vi "OEE_SCREEN_2_show_label_for_graphics.vi"(10 "Y_annotation_offset":dbl, 11 "values":cluster{dbl[], dbl[]}) -> (3 "annotations":T1(array[cluster]))   [LabVIEW 2020]
uses:
  <vilib>/Analysis/baseanly.llb/Mean (DBL).vi
  <vilib>/Analysis/NI_AALBase.lvlib
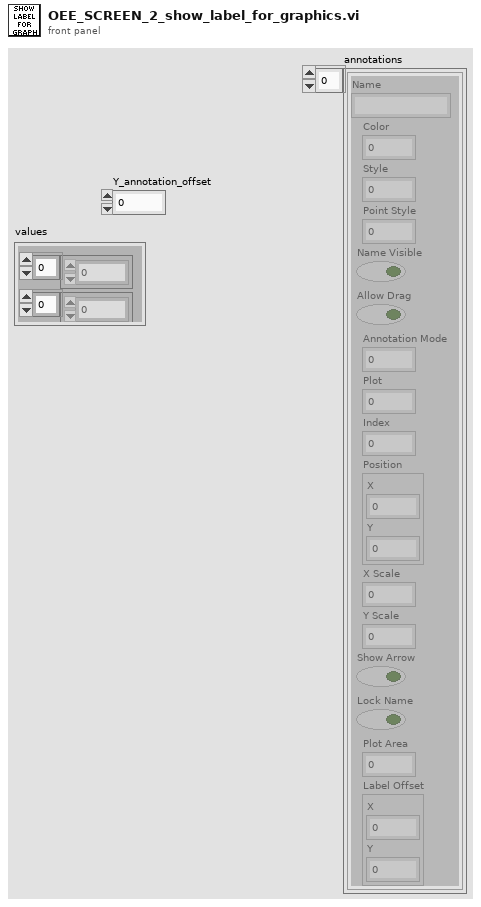
[diagram p1: front panel]
types:
  T1 = cluster{"Name":string, "Color":u32, "Style":u8, "Point Style":u8, "Name Visible":bool, "Allow Drag":bool, "Annotation Mode":u32, "Plot":i32, "Index":i32, "Position":cluster{"X":dbl, "Y":dbl}, "X Scale":u32, "Y Scale":u32, "Show Arrow":bool, "Lock Name":bool, "Plot Area":i32, "Label Offset":cluster{"X":dbl, "Y":dbl}}[]
  T2 = cluster{"Name":string, "Color":u32, "Style":u8, "Point Style":u8, "Name Visible":bool, "Allow Drag":bool, "Annotation Mode":u32, "Plot":i32, "Index":i32, "Position":cluster{"X":dbl, "Y":dbl}, "X Scale":u32, "Y Scale":u32, "Show Arrow":bool, "Lock Name":bool, "Plot Area":i32, "Label Offset":cluster{"X":dbl, "Y":dbl}}
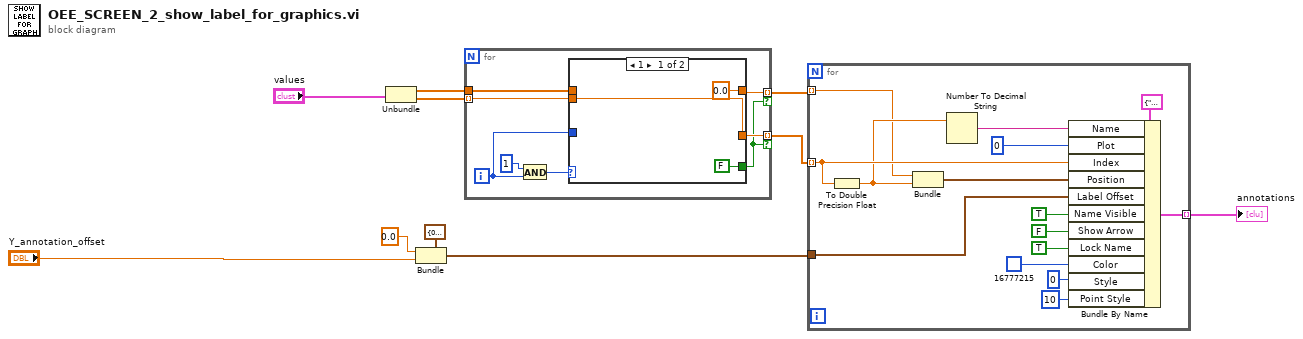
[diagram p0: block diagram]
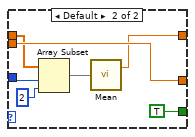
[diagram p2: hidden frame]
diagram:
  n1 = Unbundle("values") -> (w5:dbl[], w4:dbl[])
  n2 = Bundle(cluster=cluster{dbl, dbl} {0.0, 0.0} ("Annotation Offset"), 0.0, "Y_annotation_offset") -> (w8:cluster{dbl, dbl})
  n3 = for {
    tunnel: w5 -> [w13]
    tunnel: w4 -> [w15] mode=indexing
    tunnel: [w14] -> w2 mode=indexing if=w12
    tunnel: [w11] -> w3 mode=indexing if=w12
    i -> [w16]
    n4 = And(x=1, y=w16) -> (x .and. y?=w17:i32)
    n5 = case shown="1" w17 {
      tunnel: w16 -> [_ w24]
      tunnel: [FALSE TRUE] -> w12
      tunnel: w15 -> [w20 w27]
      tunnel: [w20 w27] -> w14
      tunnel: w13 -> [_ w26]
      tunnel: [0.0 ("mean") w22] -> w11
      frame 1 {
      }
      frame Default {
        n6 = Array Subset(array=w26, index=w24, length=2) -> (w25:dbl[])
        n7 = call-poly <vilib>:"Mean.vi"("X"=w25) -> ("mean"=w22:dbl)  [unwired: 1 out]
      }
    }
  }
  n8 = for {
    tunnel: w2 -> [w36] mode=indexing
    tunnel: [w38] -> w6 mode=indexing
    tunnel: w3 -> [w31] mode=indexing
    tunnel: w8 -> [w29]
    n9 = To Double Precision Float(number=w36) -> (double precision float=w32:dbl)
    n10 = Bundle("mean"=w31, w32) -> (w33:cluster{"mean":dbl, dbl})  [unwired: 1 in]
    n11 = Number To Decimal String(number=w32) -> (decimal integer string=w42:string)  [unwired: 1 in]
    n12 = Bundle By Name(cluster=T2 {"Name"="", "Color"=0, "Style"=0, "Point Style"=0, "Name Visible"=FALSE, "Allow Drag"=FALSE, "Annotation Mode"=0, "Plot"=0, "Index"=0, "Position"={"X"=0.0, "Y"=0.0}, "X Scale"=0, "Y Scale"=0, "Show Arrow"=FALSE, "Lock Name"=FALSE, "Plot Area"=0, "Label Offset"={"X"=0.0, "Y"=0.0}}, "Name"=w42, "Plot"=0, "Index"=w36, "Position"=w33, "Label Offset"=w29, "Name Visible"=TRUE, "Show Arrow"=FALSE, "Lock Name"=TRUE, "Color"=u32 16777215, "Style"=u8 0, "Point Style"=u8 10) -> (w38:T2)
  }
  "annotations" <- w6
